vi "RSD Msg Send To Router.vi"(8 "error in (no error)":errorcluster, 10 "RDS Message":refnum<class "RDS Message.lvclass">, 11 "RDS Router Actor in":refnum<class "RDS Router Actor.lvclass">) -> (0 "error out":errorcluster, 3 "RDS Router Actor out":refnum<class "RDS Router Actor.lvclass">)   [LabVIEW 2015, in "RDS Abstracts.lvlib" / "RDS Router Actor.lvlib" / "RDS Router Actor.lvclass"]
uses:
  RDS Router Actor.lvclass
  Libraries/RDS Framework/RDS Message Class/RDS Message.lvclass
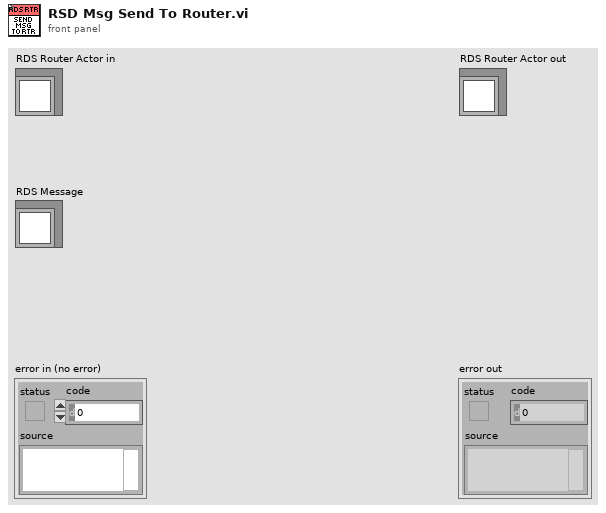
[diagram p1: front panel]
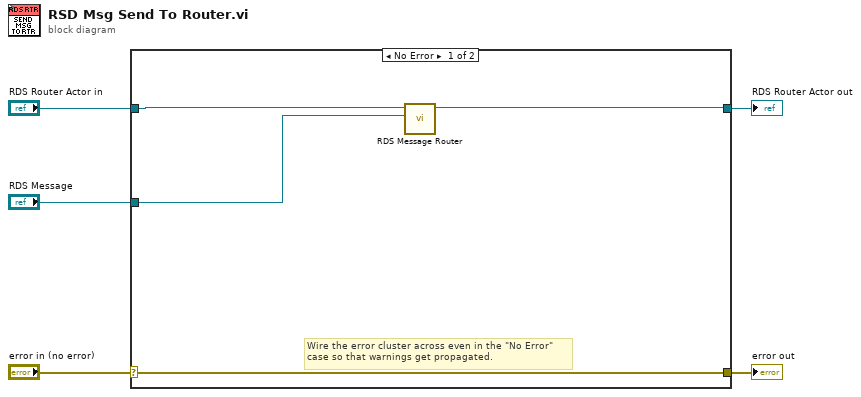
[diagram p0: block diagram]
diagram:
  n1 = case shown="No Error" "error in (no error)" {
    selector: "error in (no error)" -> [w9 w11]
    tunnel: [w9 w11] -> w4
    tunnel: [w7 w10] -> w2
    tunnel: "RDS Router Actor in" -> [w8 w10]
    tunnel: "RDS Message" -> [w6 _]
    frame No Error {
      # "Wire the error cluster across even in the \"No Error\"\ncase so that warnings get propagated."
      n2 = call "RDS Message Router.vi"("RDS Message"=w6, "RDS Router Actor in"=w8) -> ("RDS Router Actor out"=w7:refnum<class "RDS Router Actor.lvclass">)  [unwired: 8 in, 1 out]
    }
    frame Error {
    }
  }
  "error out" <- w4
  "RDS Router Actor out" <- w2
